vi "Update Load Forecast Longterm.vi"(10 "Load Power Forecast":T1, 11 "Optimization in":refnum<class "Optimization.lvclass">) -> (3 "Optimization out":refnum<class "Optimization.lvclass">)   [LabVIEW 2016, in "Optimization Framework.lvlib" / "Optimization.lvclass"]
uses:
  Optimization.lvclass
  Controls/Forecast Device Power.ctl
  Controls/PDF Cluster.ctl
  Optimization.lvclass/Optimization.ctl
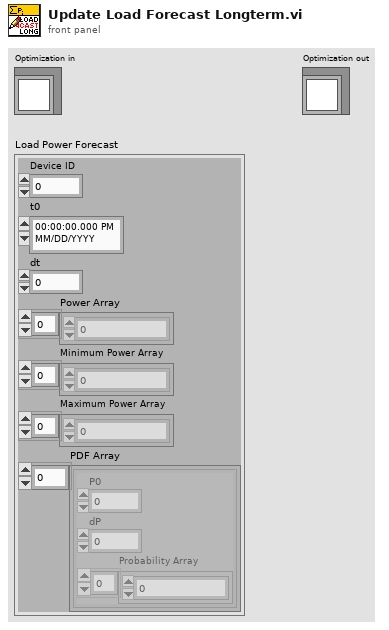
[diagram p1: front panel]
types:
  T1 = typedef "Optimization Framework.lvlib/Optimization.lvclass/Forecast Device Power.ctl" = cluster{"Device ID":u64, "t0":timestamp, "dt":dbl, "Power Array":dbl[], "Minimum Power Array":dbl[], "Maximum Power Array":dbl[], "PDF Array":T2[]}
  T2 = typedef "Optimization Framework.lvlib/Optimization.lvclass/PDF Cluster.ctl" = cluster{"P0":dbl, "dP":dbl, "Probability Array":dbl[]}
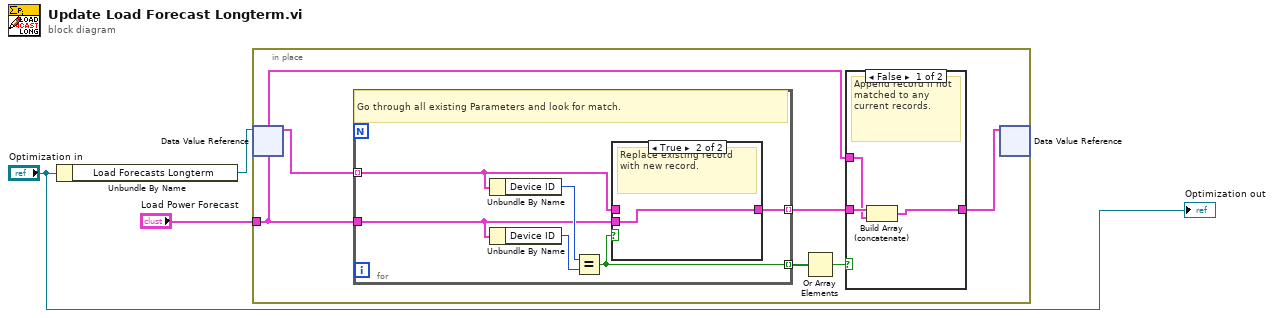
[diagram p0: block diagram]
diagram:
  n1 = Unbundle By Name("Optimization in") -> ("Load Forecasts Longterm"=w1:refnum<data-value>)
  n2 = in-place {
    in-place-border: "Load Power Forecast" -> [w6]
    n3 = in-place-dvr #1(w1) -> (w4:T1[])  [unwired: 1 out]
    n4 = for {
      tunnel: w4 -> [w15] mode=indexing
      tunnel: w6 -> [w16]
      tunnel: [w17] -> w9 mode=indexing
      tunnel: [w14] -> w7 mode=indexing
      # "Go through all existing Parameters and look for match."
      n5 = Unbundle By Name(w15) -> ("Device ID"=w19:u64)
      n6 = Unbundle By Name(w16) -> ("Device ID"=w18:u64)
      n7 = Equal?(x=w19, y=w18) -> (x = y?=w14:bool)
      n8 = case shown="True" w14 {
        tunnel: [w20 w21] -> w17
        tunnel: w16 -> [_ w21]
        tunnel: w15 -> [w20 _]
        frame False {
          # "Keep existing record."
        }
        frame True {
          # "Replace existing record with new record."
        }
      }
    }
    n9 = Or Array Elements(Boolean array=w7) -> (logical OR=w8:bool)
    n10 = case shown="False" w8 {
      tunnel: w6 -> [w11 _]
      tunnel: w9 -> [w12 w13]
      tunnel: [w10 w13] -> w5
      frame False {
        # "Append record if not matched to any current records."
        n11 = Build Array (concatenate)(w12, w11) -> (w10:T1[])
      }
      frame True {
        # "Record was replaced, pass through."
      }
    }
    n12 = in-place-dvr #1(w5) -> ()  [unwired: 2 out]
  }
  "Optimization out" <- "Optimization in"
